vi "cm2nm_pair_fiducicials_fromData.vi"(0 "CurrentSessionDataSet":T1[](array[typedef])=[{"MetaDataFile"=path "", "X"=1.1, "Y"=0.0, "Z"=0.0, "Group"=0, "Rotation"=0.0, "Fiducial"=TRUE, "Magnification"=0.0, "Working_Distance"=0.0, "Notes"="", "Location Name/ID"="", "OtherRelatedDataFiles"=[], "Available"=FALSE}, {"MetaDataFile"=path "", "X"=0.0, "Y"=1.0, "Z"=0.0, "Group"=0, "Rotation"=0.0, "Fiducial"=TRUE, "Magnification"=0.0, "Working_Distance"=0.0, "Notes"="", "Location Name/ID"="", "OtherRelatedDataFiles"=[], "Available"=FALSE}, {"MetaDataFile"=path "", "X"=0.0, "Y"=-1.0, "Z"=0.0, "Group"=0, "Rotation"=0.0, "Fiducial"=TRUE, "Magnification"=0.0, "Working_Distance"=0.0, "Notes"="", "Location Name/ID"="", "OtherRelatedDataFiles"=[], "Available"=FALSE}, {"MetaDataFile"=path "", "X"=-1.0, "Y"=0.0, "Z"=0.0, "Group"=0, "Rotation"=0.0, "Fiducial"=TRUE, "Magnification"=0.0, "Working_Distance"=0.0, "Notes"="", "Location Name/ID"="", "OtherRelatedDataFiles"=[], "Available"=FALSE}, {"MetaDataFile"=path "", "X"=0.0, "Y"=0.0, "Z"=0.0, "Group"=0, "Rotation"=0.0, "Fiducial"=TRUE, "Magnification"=0.0, "Working_Distance"=0.0, "Notes"="", "Location Name/ID"="", "OtherRelatedDataFiles"=[], "Available"=FALSE}], 1 "ReferenceSessionDataSet":T1[](array[typedef])=[{"MetaDataFile"=path "", "X"=-1.1, "Y"=0.0, "Z"=0.0, "Group"=0, "Rotation"=0.0, "Fiducial"=TRUE, "Magnification"=0.0, "Working_Distance"=0.0, "Notes"="", "Location Name/ID"="", "OtherRelatedDataFiles"=[], "Available"=FALSE}, {"MetaDataFile"=path "", "X"=0.0, "Y"=-1.0, "Z"=0.0, "Group"=0, "Rotation"=0.0, "Fiducial"=TRUE, "Magnification"=0.0, "Working_Distance"=0.0, "Notes"="", "Location Name/ID"="", "OtherRelatedDataFiles"=[], "Available"=FALSE}, {"MetaDataFile"=path "", "X"=0.0, "Y"=1.0, "Z"=0.0, "Group"=0, "Rotation"=0.0, "Fiducial"=TRUE, "Magnification"=0.0, "Working_Distance"=0.0, "Notes"="", "Location Name/ID"="", "OtherRelatedDataFiles"=[], "Available"=FALSE}, {"MetaDataFile"=path "", "X"=1.0, "Y"=0.0, "Z"=0.0, "Group"=0, "Rotation"=0.0, "Fiducial"=TRUE, "Magnification"=0.0, "Working_Distance"=0.0, "Notes"="", "Location Name/ID"="", "OtherRelatedDataFiles"=[], "Available"=FALSE}], 4 "UseBestFit":bool) -> (2 "CurrentSessionOut":T1[](array[typedef])=[{"MetaDataFile"=path "", "X"=-1.1, "Y"=0.0, "Z"=0.0, "Group"=0, "Rotation"=0.0, "Fiducial"=TRUE, "Magnification"=0.0, "Working_Distance"=0.0, "Notes"="", "Location Name/ID"="", "OtherRelatedDataFiles"=[], "Available"=FALSE}, {"MetaDataFile"=path "", "X"=0.0, "Y"=-1.0, "Z"=0.0, "Group"=0, "Rotation"=0.0, "Fiducial"=TRUE, "Magnification"=0.0, "Working_Distance"=0.0, "Notes"="", "Location Name/ID"="", "OtherRelatedDataFiles"=[], "Available"=FALSE}, {"MetaDataFile"=path "", "X"=0.0, "Y"=1.0, "Z"=0.0, "Group"=0, "Rotation"=0.0, "Fiducial"=TRUE, "Magnification"=0.0, "Working_Distance"=0.0, "Notes"="", "Location Name/ID"="", "OtherRelatedDataFiles"=[], "Available"=FALSE}, {"MetaDataFile"=path "", "X"=1.0, "Y"=0.0, "Z"=0.0, "Group"=0, "Rotation"=0.0, "Fiducial"=TRUE, "Magnification"=0.0, "Working_Distance"=0.0, "Notes"="", "Location Name/ID"="", "OtherRelatedDataFiles"=[], "Available"=FALSE}], 3 "Best_fit_and_name_match.":bool, 5 "BestFitDistance":dbl, 6 "EnoughmatchingFiducials":bool, 7 "PairedFiducialNames":T2(array[cluster]), 8 "PairedFiducials":T3(array[cluster])=[{"X1"=1.1, "X2"=-1.1, "Y1"=0.0, "Y2"=0.0, "Z1"=0.0, "Z2"=0.0}, {"X1"=0.0, "X2"=0.0, "Y1"=1.0, "Y2"=-1.0, "Z1"=0.0, "Z2"=0.0}, {"X1"=0.0, "X2"=0.0, "Y1"=-1.0, "Y2"=1.0, "Z1"=0.0, "Z2"=0.0}, {"X1"=-1.0, "X2"=1.0, "Y1"=0.0, "Y2"=0.0, "Z1"=0.0, "Z2"=0.0}], 9 "NumberOfNameMatch":i32, 10 "OK_num_fids?":bool)   [LabVIEW 2011]
doc: "Routine populates the structure for paired fiducials between the reference and current sessions for use in calculating the transformation matrix. The routine also performs an diagnostic check to find the best geometrical fit between the two sets of fiducials."
uses:
  cm2nm_coordinate_information_v2.ctl
panel:
  out "CurrentSessionFitIndex":i32[](array[numeric])
  out "Matched_Fiducail_Index_Reference_byName":i32[](array[numeric])
  out "Matched_Fiducial_Index_Current_byName":i32[](array[numeric])
  out "ReferenceIndex":i32[](array[numeric])
  out "Results Out":i32[][](array[numeric])
  out "IndexRefrenceSession":i32[][](array[numeric])
  out "BestFitReference":i32[](array[numeric])
  out "Index of Best Fit":i32
  out "Distances":dbl[](array[numeric])
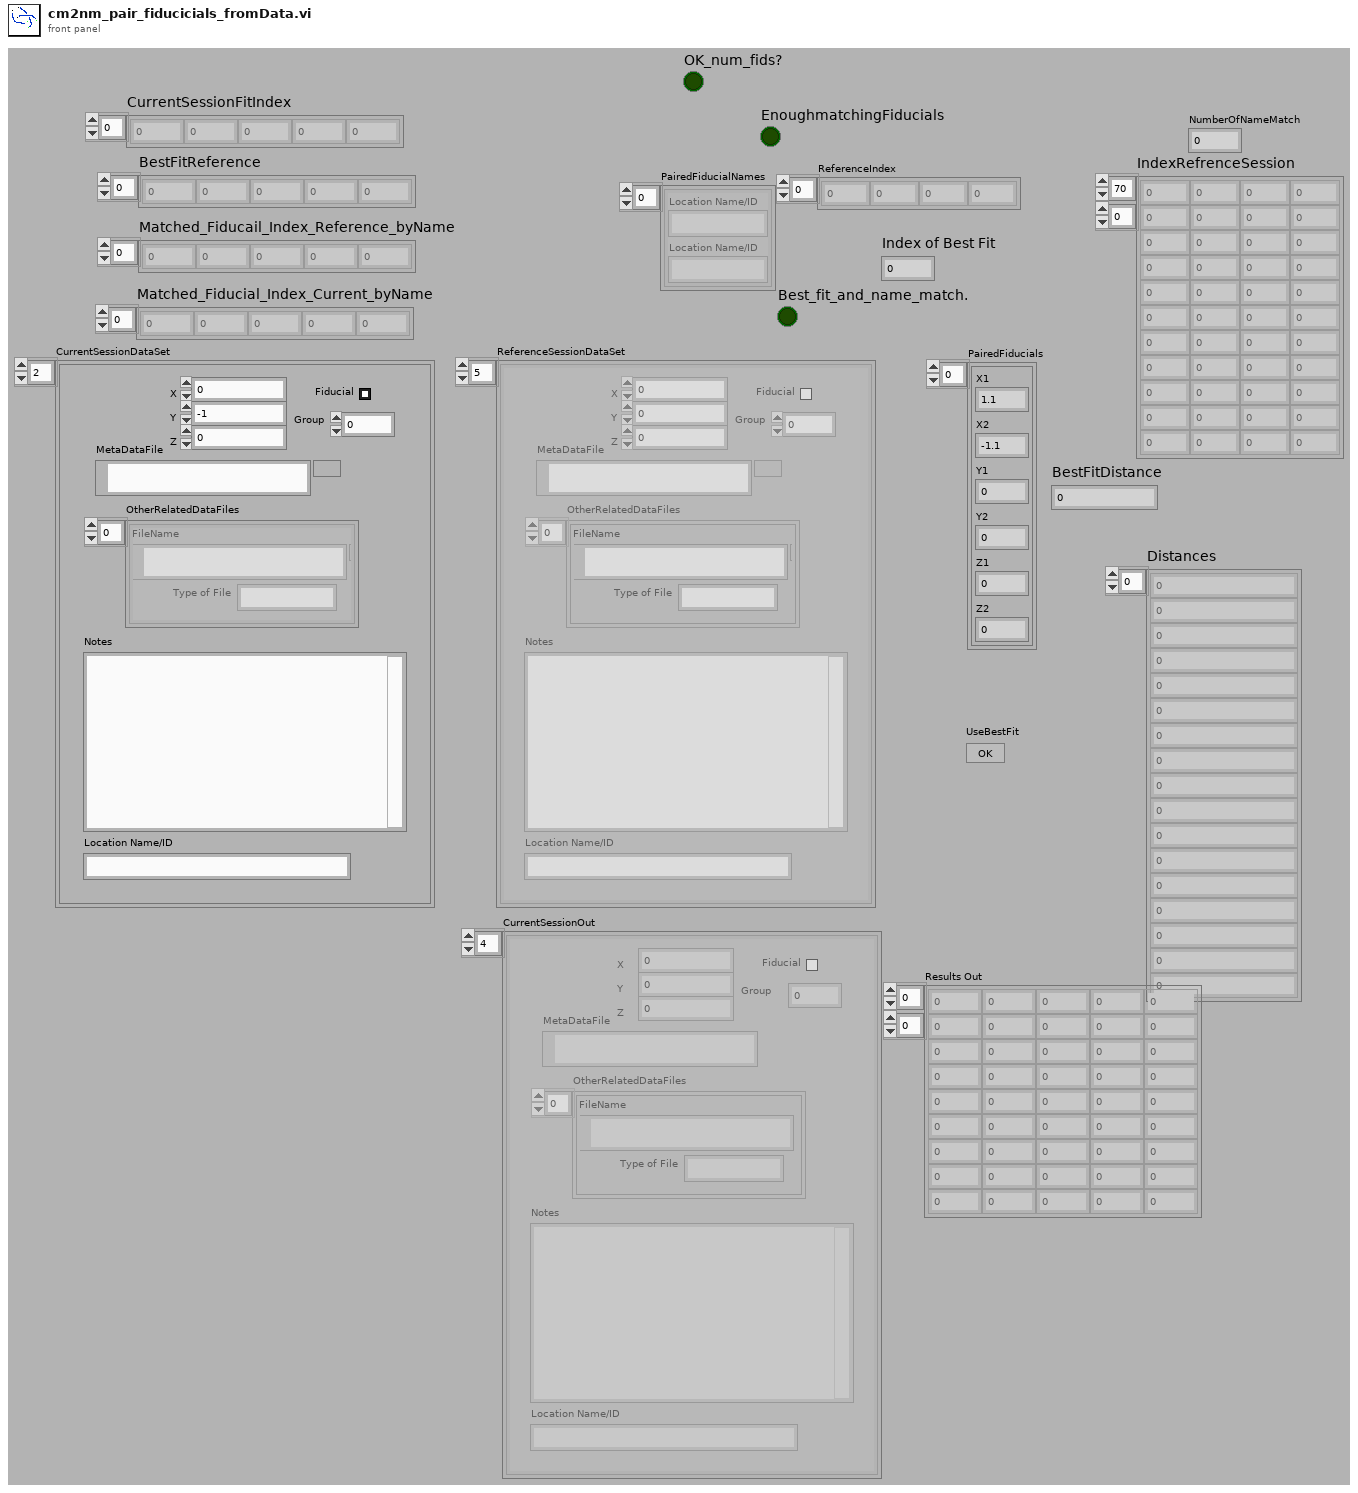
[diagram p1: front panel]
types:
  T1 = typedef "cm2nm_coordinate_information_v2.ctl" = cluster{"MetaDataFile":path, "X":dbl, "Y":dbl, "Z":dbl, "Group":i32, "Rotation":dbl[unit], "Fiducial":bool, "Magnification":dbl, "Working_Distance":dbl, "Notes":string, "Location Name/ID":string, "OtherRelatedDataFiles":cluster{"Type of File":string, "FileName":path}[], "Available":bool}
  T2 = cluster{"Location Name/ID":string, "Location Name/ID":string}[]
  T3 = cluster{"X1":dbl, "X2":dbl, "Y1":dbl, "Y2":dbl, "Z1":dbl, "Z2":dbl}[]
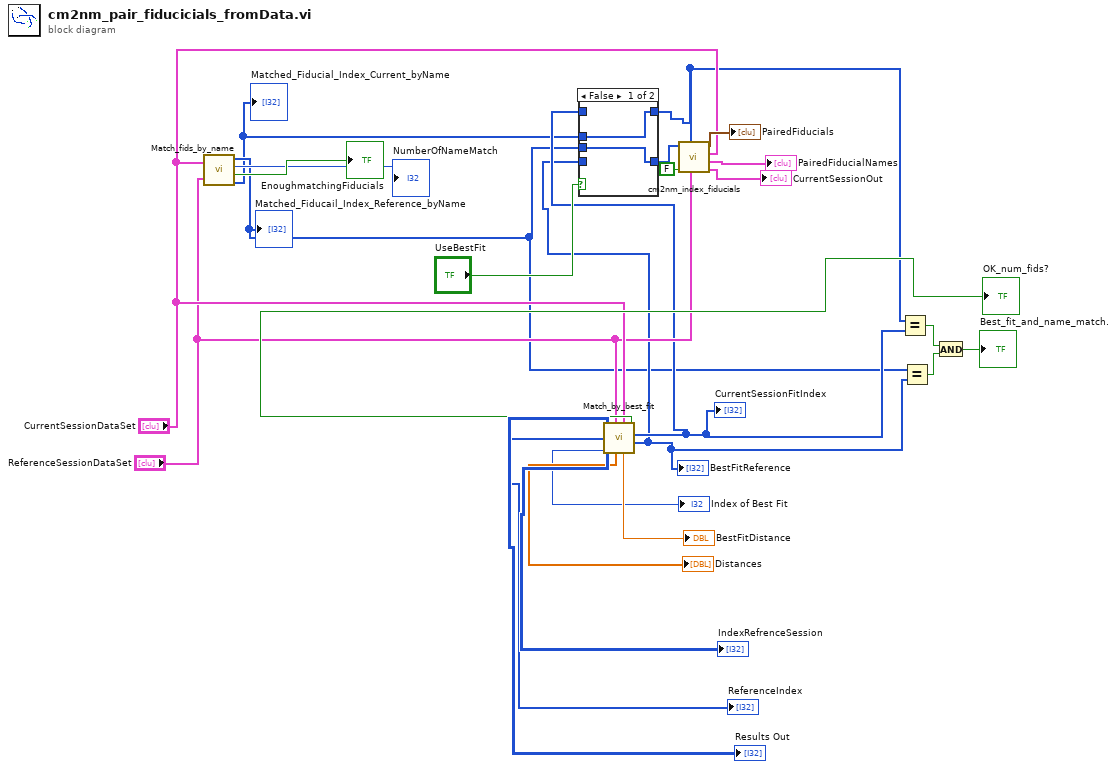
[diagram p0: block diagram]
diagram:
  n1 = call "Match_fids_by_name.vi"("CurrentSessionDataSet"="CurrentSessionDataSet", "ReferenceSessionDataSet"="ReferenceSessionDataSet") -> ("ReferenceMatch"=w2:i32[], "NumberOfNameMatch"=→"NumberOfNameMatch":i32, "AtLeast3"=→"EnoughmatchingFiducials":bool, "CurrentMatch"=w1:i32[])
  "Matched_Fiducial_Index_Current_byName" <- w1
  "Matched_Fiducail_Index_Reference_byName" <- w2
  n2 = call "Match_by_best_fit.vi"("ReferenceSessionDataSet"="ReferenceSessionDataSet", "CurrentSessionDataSet"="CurrentSessionDataSet") -> ("Results Out"=→"Results Out":i32[][], "Array"=→"ReferenceIndex":i32[], "IndexRefrenceSession 3"=→"IndexRefrenceSession":i32[][], "Array 2"=→"Distances":dbl[], "Boolean"=→"OK_num_fids?":bool, "IndexRefrenceSession"=w7:i32[], "Numeric 2"=→"BestFitDistance":dbl, "IndexRefrenceSession 2"=w5:i32[], "Numeric"=→"Index of Best Fit":i32)
  "BestFitReference" <- w5
  "CurrentSessionFitIndex" <- w7
  n3 = case shown="False" "UseBestFit" {
    tunnel: w7 -> [_ w29]
    tunnel: [w26 w29] -> w6
    tunnel: w5 -> [_ w28]
    tunnel: [w27 w28] -> w4
    tunnel: w2 -> [w27 _]
    tunnel: w1 -> [w26 _]
    frame False {
    }
    frame True {
    }
  }
  n4 = call "cm2nm_index_fiducials.vi"("CurrentSessionCollectionOfPoints"="CurrentSessionDataSet", "ReferenceSessionCollectionOfPoints"="ReferenceSessionDataSet", "IndexCurrentSession_PairingList"=w6, "ReplacePairedFidName"=FALSE, "IndexRefrenceSession_PairlingList"=w4) -> ("CurrentSessionOut"=→"CurrentSessionOut":T1[], "PairedFiducialNames"=→"PairedFiducialNames":T2, "PairedFiducials"=→"PairedFiducials":T3)  [unwired: 2 in]
  n5 = Equal?(x=w6, y=w7) -> (x = y?=w11:bool)
  n6 = Equal?(x=w2, y=w5) -> (x = y?=w12:bool)
  n7 = And(x=w11, y=w12) -> (x .and. y?=→"Best_fit_and_name_match.":bool)
